vi "Test Serialize Enum.vi"(8 "error in (no error)":errorcluster) -> (0 "error out":errorcluster)   [LabVIEW 2013]
uses:
  src/Serializer/JSON Serializer/JSON Serializer.lvclass
  <vilib>/addons/_JKI Toolkits/Caraya/classes/Test/Test.lvclass
  <vilib>/addons/_JKI Toolkits/Caraya/classes/Assert/Assert.lvclass
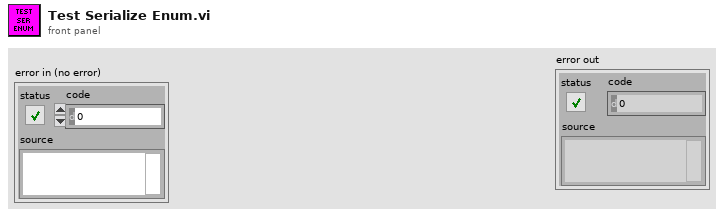
[diagram p1: front panel]
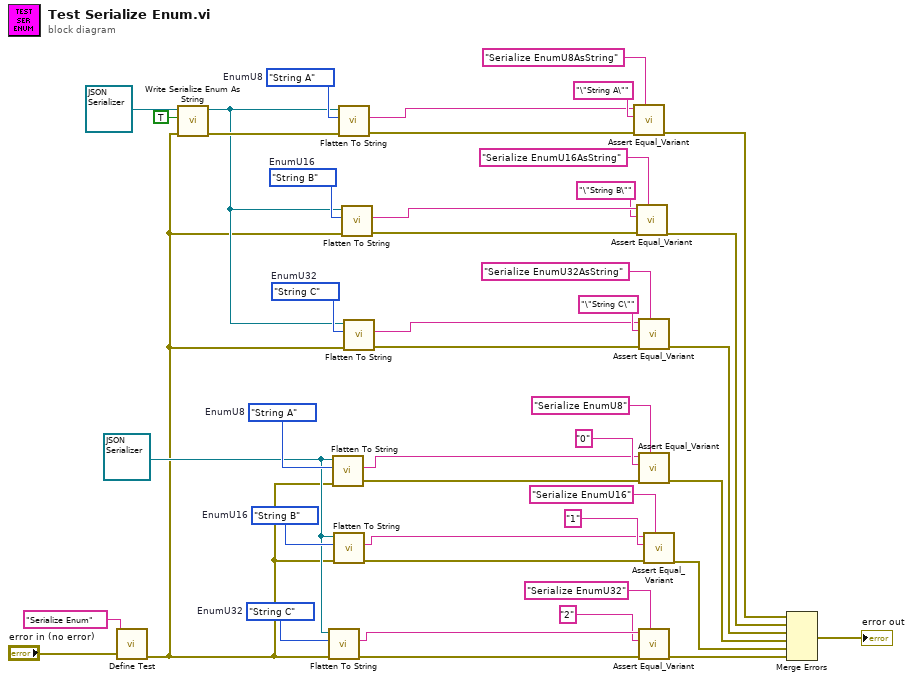
[diagram p0: block diagram]
diagram:
  w9 = enum32{"String A", "String B", "String C"}."String C"  # EnumU32
  w10 = enum16{"String A", "String B", "String C"}."String B"  # EnumU16
  w15 = refnum<class "JSON Serializer.lvclass"> refnum ("JKI JSON Serialization.lvlib:JSON Serializer.lvclass")
  w23 = enum8{"String A", "String B", "String C"}."String A"  # EnumU8
  w30 = enum16{"String A", "String B", "String C"}."String B"  # EnumU16
  w32 = enum32{"String A", "String B", "String C"}."String C"  # EnumU32
  w33 = enum8{"String A", "String B", "String C"}."String A"  # EnumU8
  n1 = call <vilib>:"Define Test.vi"("error in (no error)"="error in (no error)", "Label (VI Title)"="Serialize Enum") -> ("error out"=w1:errorcluster)  [unwired: 9 in]
  n2 = call-dynamic "Write Serialize Enum As String.vi"("error in (no error)"=w1, "Enums As String"=TRUE ("enumAsString"), "JSON Serializer in"=refnum<class "JSON Serializer.lvclass"> refnum ("JKI JSON Serialization.lvlib:JSON Serializer.lvclass")) -> ("error out"=w18:errorcluster, "JSON Serializer out"=w2:refnum<class "JSON Serializer.lvclass">)  [unwired: 7 in]
  n3 = call-dynamic "Flatten To String.vi"("error in (no error)"=w1, "Variant"=w32, "JSON Serializer in"=w15) -> ("error out"=w43:errorcluster, "String"=w41:string)  [unwired: 6 in, 1 out]
  n4 = call-dynamic "Flatten To String.vi"("error in (no error)"=w1, "Variant"=w33, "JSON Serializer in"=w15) -> ("error out"=w36:errorcluster, "String"=w35:string)  [unwired: 6 in, 1 out]
  n5 = call-dynamic "Flatten To String.vi"("error in (no error)"=w1, "Variant"=w30, "JSON Serializer in"=w15) -> ("error out"=w26:errorcluster, "String"=w27:string)  [unwired: 6 in, 1 out]
  n6 = call-dynamic "Flatten To String.vi"("error in (no error)"=w18, "Variant"=w23, "JSON Serializer in"=w2) -> ("error out"=w19:errorcluster, "String"=w20:string)  [unwired: 6 in, 1 out]
  n7 = call-dynamic "Flatten To String.vi"("error in (no error)"=w1, "Variant"=w10, "JSON Serializer in"=w2) -> ("error out"=w14:errorcluster, "String"=w13:string)  [unwired: 6 in, 1 out]
  n8 = call-dynamic "Flatten To String.vi"("error in (no error)"=w1, "Variant"=w9, "JSON Serializer in"=w2) -> ("error out"=w5:errorcluster, "String"=w6:string)  [unwired: 6 in, 1 out]
  n9 = call <vilib>:"Assert Equal_Variant.vi"("Label"="Serialize EnumU8AsString", "error in (no error)"=w19, "Y"="\"String A\"", "X"=w20) -> ("error out"=w16:errorcluster)  [unwired: 7 in]
  n10 = call <vilib>:"Assert Equal_Variant.vi"("Label"="Serialize EnumU16AsString", "error in (no error)"=w14, "Y"="\"String B\"", "X"=w13) -> ("error out"=w4:errorcluster)  [unwired: 7 in]
  n11 = call <vilib>:"Assert Equal_Variant.vi"("Label"="Serialize EnumU32AsString", "error in (no error)"=w5, "Y"="\"String C\"", "X"=w6) -> ("error out"=w3:errorcluster)  [unwired: 7 in]
  n12 = call <vilib>:"Assert Equal_Variant.vi"("Label"="Serialize EnumU8", "error in (no error)"=w36, "Y"="0", "X"=w35) -> ("error out"=w31:errorcluster)  [unwired: 7 in]
  n13 = call <vilib>:"Assert Equal_Variant.vi"("Label"="Serialize EnumU32", "error in (no error)"=w43, "Y"="2", "X"=w41) -> ("error out"=w42:errorcluster)  [unwired: 7 in]
  n14 = call <vilib>:"Assert Equal_Variant.vi"("Label"="Serialize EnumU16", "error in (no error)"=w26, "Y"="1", "X"=w27) -> ("error out"=w25:errorcluster)  [unwired: 7 in]
  n15 = Merge Errors(w16, w4, w3, w31, w25, w42) -> (→"error out":errorcluster)
